vi "Low Speed Mode.vi"(8 "Error in":errorcluster, 11 "section":string) -> (0 "Error out":errorcluster, 3 "This VI":refnum<vi>)   [LabVIEW 2020]
uses:
  <vilib>/Utility/config.llb/Read Key (Double).vi
  <vilib>/Utility/config.llb/NI_LVConfig.lvlib
panel:
  out "Clock Frequency":dbl format="%#_g kHz"
  out "T hd:sta":dbl format="%#_g µs"
  out "T low":dbl format="%#_g µs"
  out "T high":dbl format="%#_g µs"
  out "T su:sta":dbl format="%#_g µs"
  out "T hd:dat":dbl format="%#_g µs"
  out "T su:dat":dbl format="%#_g ns"
  out "T su:sto":dbl format="%#_g µs"
  out "T buf":dbl format="%#_g µs"
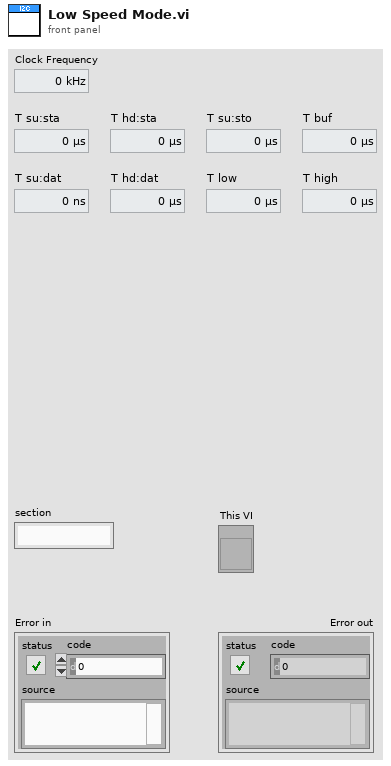
[diagram p1: front panel]
types:
  T1 = typedef "NI_LVConfig.lvlib/Config Data RefNum.ctl" = refnum<k1>
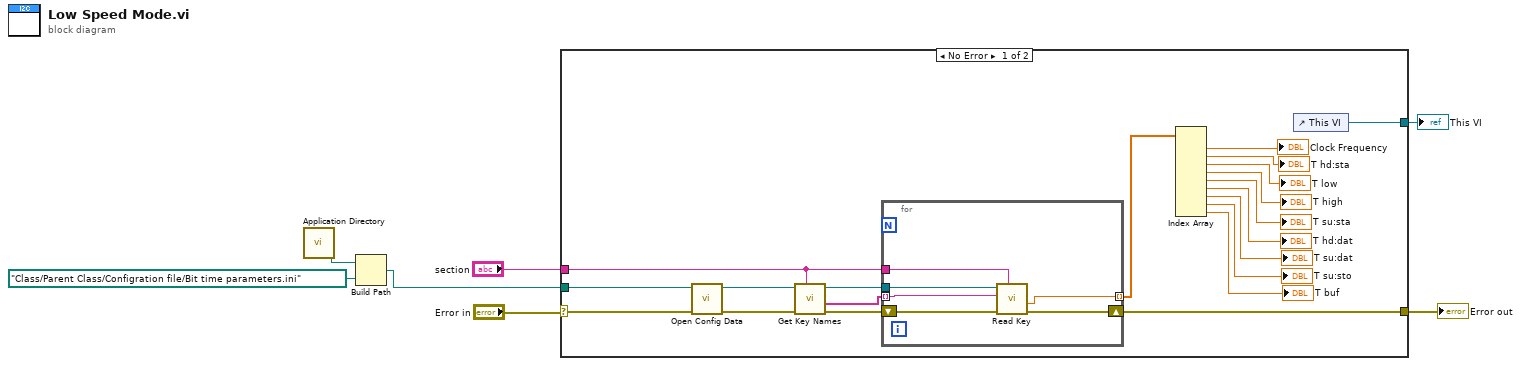
[diagram p0: block diagram]
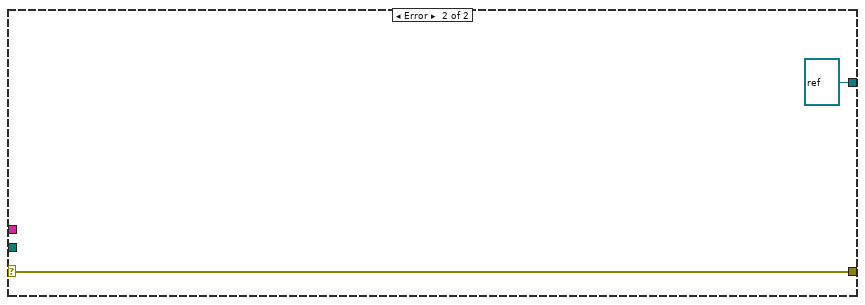
[diagram p2: hidden frame]
diagram:
  n1 = call <vilib>:"Application Directory.vi"() -> ("Application Directory"=w7:path)
  n2 = Build Path(base path=w7, name or relative path=path "Class/Parent Class/Configration file/Bit time parameters.ini") -> (appended path=w2:path)
  n3 = case shown="No Error" "Error in" {
    selector: "Error in" -> [w25 w35]
    tunnel: [w23 w35] -> w4
    tunnel: "section" -> [w21 _]
    tunnel: w2 -> [w9 _]
    tunnel: [w8 refnum<vi> refnum ("This VI")] -> w1
    frame No Error {
      n4 = call <vilib>:"Open Config Data.vi"("error in (no error)"=w25, "configuration file path"=w9) -> ("error out"=w27:errorcluster, "refnum"=w26:T1)  [unwired: 7 in, 1 out]
      n5 = call <vilib>:"Get Key Names.vi"("section"=w21, "error in (no error)"=w27, "refnum"=w26) -> ("error out"=w24:errorcluster, "key names"=w20:string[], "refnum out"=w22:T1)  [unwired: 5 in, 1 out]
      n6 = for {
        tunnel: w22 -> [w31]
        tunnel: w21 -> [w30]
        shift-right: [w32] -> w23
        shift-left: w24 -> [w33]
        tunnel: w20 -> [w29] mode=indexing
        tunnel: [w28] -> w19 mode=indexing
        n7 = call-poly <vilib>:"Read Key.vi"("section"=w30, "error in (no error)"=w33, "key"=w29, "refnum"=w31) -> ("error out"=w32:errorcluster, "value"=w28:dbl)  [unwired: 4 in, 2 out]
      }
      n8 = Index Array(array=w19) -> (element #1=→"Clock Frequency":dbl, element #2=→"T hd:sta":dbl, element #3=→"T low":dbl, element #4=→"T high":dbl, element #5=→"T su:sta":dbl, element #6=→"T hd:dat":dbl, element #7=→"T su:dat":dbl, element #8=→"T su:sto":dbl, element #9=→"T buf":dbl)  [unwired: 9 in]
      n9 = control-ref of="This VI"() -> (w8:refnum<vi>)
    }
    frame Error {
    }
  }
  "Error out" <- w4
  "This VI" <- w1
